vi "Find Signal Parameters.vi"(11 "Worksheet Data":string[][](array[string])) -> (1 "Signal Parameter Row Index":i32, 2 "Signal Parameters":string[](array[string]), 3 "Worksheet Data Out":string[][](array[string]))   [LabVIEW 2016, in "TSF Parser.lvlib" / "TSF Parser.lvclass"]
uses:
  TSF Parser.lvclass
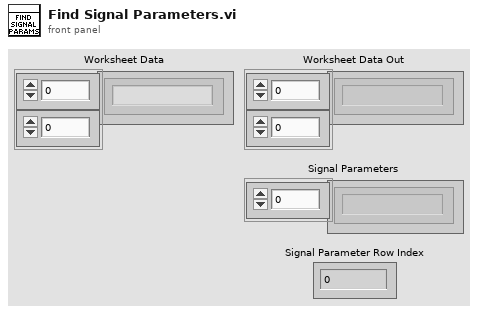
[diagram p1: front panel]
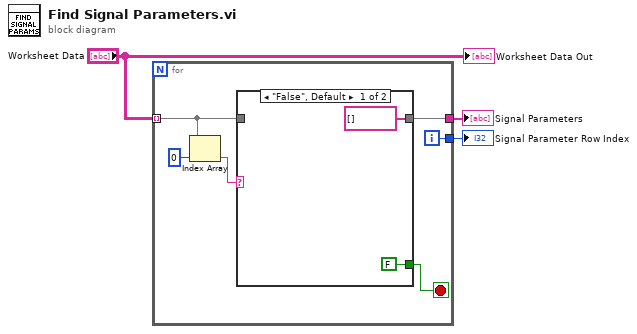
[diagram p0: block diagram]
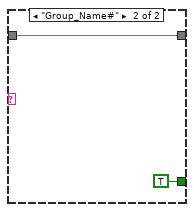
[diagram p2: hidden frame]
diagram:
  n1 = for {
    tunnel: "Worksheet Data" -> [w6] mode=indexing
    tunnel: [w5] -> w2
    tunnel: [w4] -> w1
    i -> [w4]
    stop <- w7 stop-if-true
    n2 = Index Array(array=w6, index=0) -> (element=w8:string)
    n3 = case shown="\"False\", Default" w8 {
      tunnel: [FALSE TRUE] -> w7
      tunnel: [string[] [] ("Worksheet Data") w12] -> w5
      tunnel: w6 -> [_ w12]
      frame "False", Default {
      }
      frame "Group_Name#" {
      }
    }
  }
  "Signal Parameters" <- w2
  "Signal Parameter Row Index" <- w1
  "Worksheet Data Out" <- "Worksheet Data"
